vi "Read Bool Data Filter Array.vi"(8 "error in (no error)":errorcluster, 11 "Function in":refnum<class "Function.lvclass">) -> (0 "error out":errorcluster, 2 "Bool Data Filter Array":bool[](array[boolean]), 3 "Function out":refnum<class "Function.lvclass">)   [LabVIEW 2016, in "Function Actor.lvlib" / "Function.lvclass"]
uses:
  <userlib>/Common Components/Function Actor/Function.lvclass
  <userlib>/Common Components/Function Actor/Function.lvclass/Function.ctl
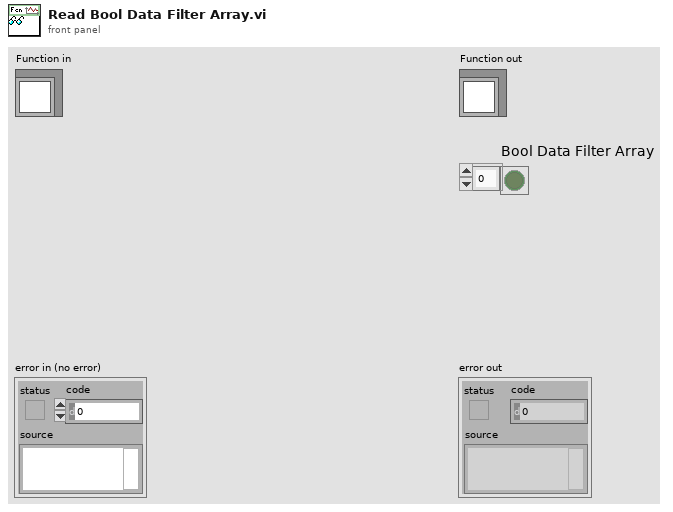
[diagram p1: front panel]
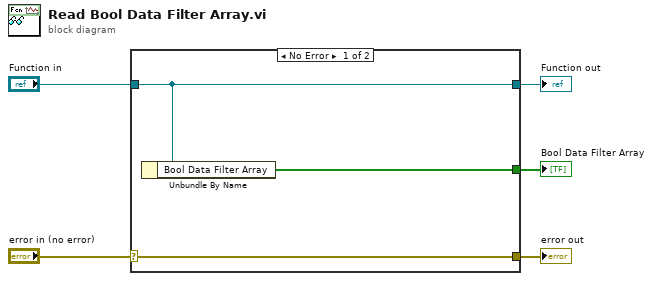
[diagram p0: block diagram]
diagram:
  n1 = case shown="No Error" "error in (no error)" {
    selector: "error in (no error)" -> [w8 w9]
    tunnel: [w8 w9] -> w4
    tunnel: [w7 w10] -> w2
    tunnel: "Function in" -> [w7 w10]
    tunnel: [w6 _] -> w1
    frame No Error {
      n2 = Unbundle By Name(w7) -> ("Bool Data Filter Array"=w6:bool[])
    }
    frame Error {
    }
  }
  "error out" <- w4
  "Function out" <- w2
  "Bool Data Filter Array" <- w1
